vi "Read Pin Map.vi"(8 "error in (no error)":errorcluster, 11 "NI-DAQ in":refnum<class "NI-DAQ.lvclass">) -> (0 "error out":errorcluster, 2 "Pin Map":T1={"Region Valves"=[49, 52, 0, 0], "Extra Valves"=[[[0.0, 48.0, 0.0, 0.0, 0.0]]], "Tool Primary Valve"=51, "Tool Secondary Valve"=50, "Region Sensors"=[37, 41, 37], "Extra Sensors"=[[[36.0, 37.0, 0.0, 0.0]]], "Tool Primary Sensor"=39.0, "Tool Secondary Sensor"=38.0, "Compression Sensor"=31.0, "5V"=50}, 3 "NI-DAQ out":refnum<class "NI-DAQ.lvclass">)   [LabVIEW 2016, in "NI-DAQ.lvclass"]
uses:
  NI-DAQ.lvclass
  Pin Map.ctl
  I-O.lvclass
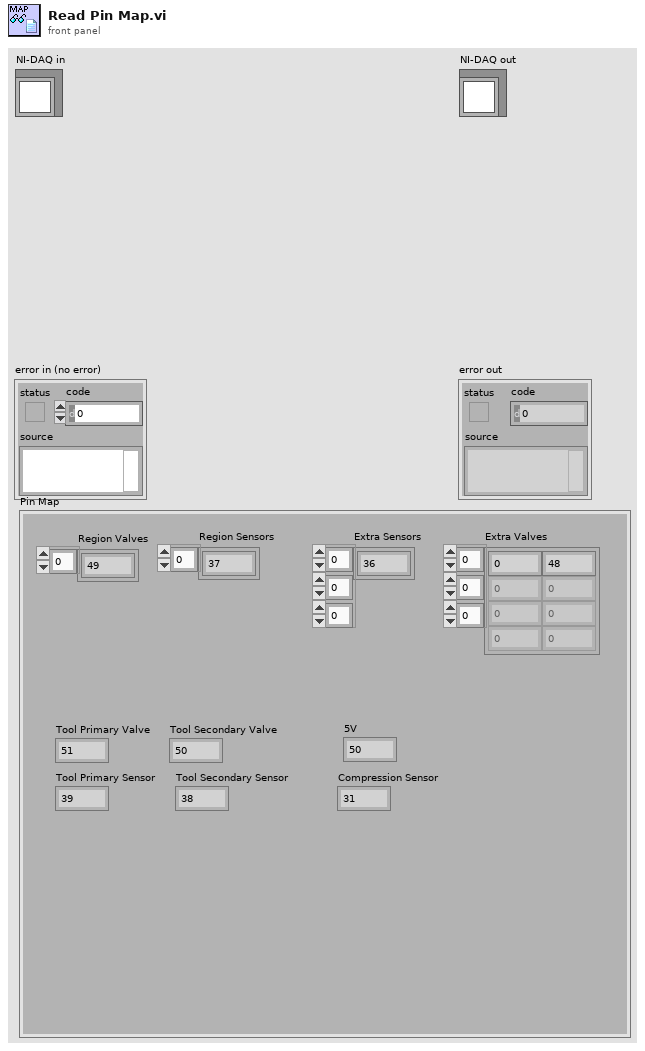
[diagram p1: front panel]
types:
  T1 = typedef "I-O.lvclass/Pin Map.ctl" = cluster{"Region Valves":i32[], "Extra Valves":dbl[][][], "Tool Primary Valve":i32, "Tool Secondary Valve":i32, "Region Sensors":i32[], "Extra Sensors":dbl[][][], "Tool Primary Sensor":dbl, "Tool Secondary Sensor":dbl, "Compression Sensor":dbl, "5V":i32}
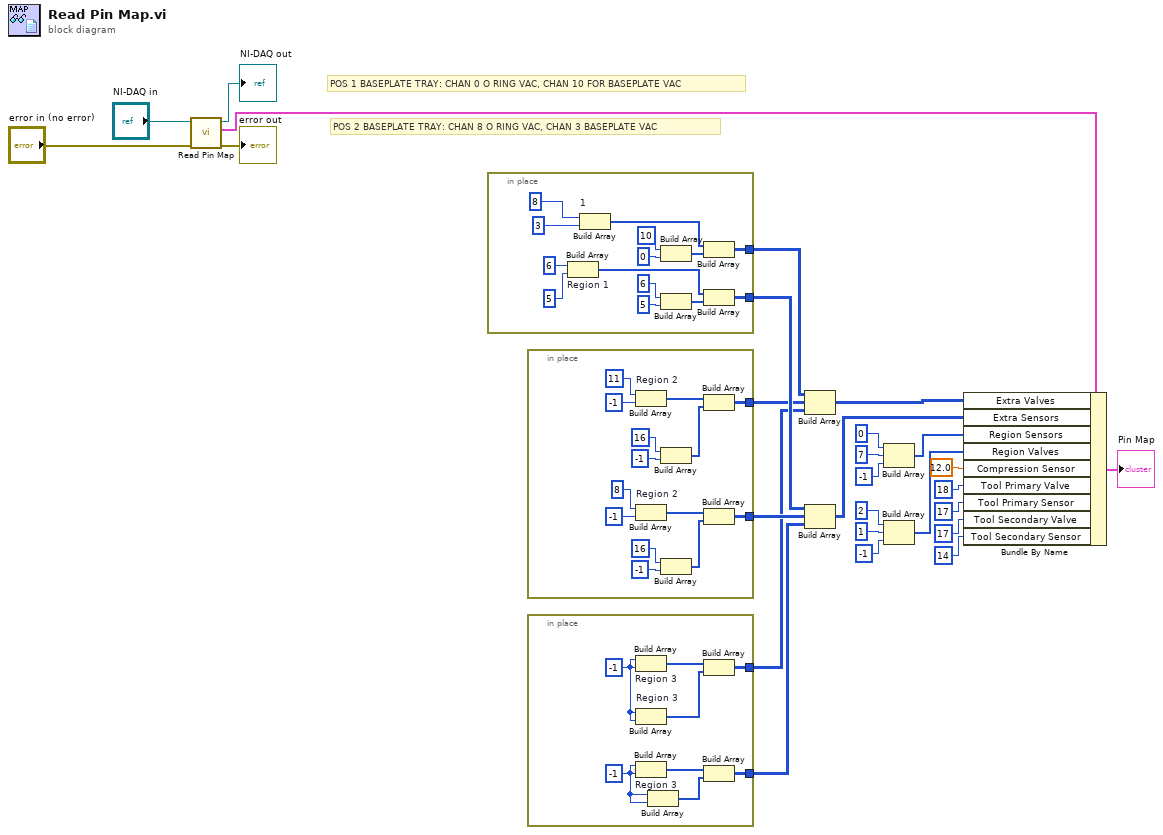
[diagram p0: block diagram]
diagram:
  # "POS 2 BASEPLATE TRAY: CHAN 8 O RING VAC, CHAN 3 BASEPLATE VAC"
  # "POS 1 BASEPLATE TRAY: CHAN 0 O RING VAC, CHAN 10 FOR BASEPLATE VAC"
  n1 = call-parent "Read Pin Map.vi"("error in (no error)"="error in (no error)", "I-O in"="NI-DAQ in") -> ("error out"=→"error out":errorcluster, "Pin Map"=w23:T1, "I-O out"=→"NI-DAQ out":refnum<class "NI-DAQ.lvclass">)  [unwired: 7 in]
  n2 = in-place {
    in-place-border: [w28] -> w8
    in-place-border: [w33] -> w3
    n3 = Build Array "Region 1"(6, 5 ("element")) -> (w30:i32[])
    n4 = Build Array "1"(8, 3 ("element")) -> (w35:i32[])
    n5 = Build Array(10, 0) -> (w34:i32[])
    n6 = Build Array(6 ("element"), 5 ("element")) -> (w29:i32[])
    n7 = Build Array(w35, w34) -> (w33:i32[][])
    n8 = Build Array(w30, w29) -> (w28:i32[][])
  }
  n9 = in-place {
    in-place-border: [w47] -> w7
    in-place-border: [w42] -> w6
    n10 = Build Array "Region 2"(11, -1) -> (w49:i32[])
    n11 = Build Array "Region 2"(8, -1 ("element")) -> (w44:i32[])
    n12 = Build Array(16 ("element"), -1) -> (w48:i32[])
    n13 = Build Array(16, -1 ("element")) -> (w43:i32[])
    n14 = Build Array(w49, w48) -> (w47:i32[][])
    n15 = Build Array(w44, w43) -> (w42:i32[][])
  }
  n16 = in-place {
    in-place-border: [w56] -> w5
    in-place-border: [w60] -> w4
    w59 = -1
    w63 = -1
    n17 = Build Array "Region 3"(w63, w63) -> (w62:i32[])
    n18 = Build Array "Region 3"(w63, w63) -> (w61:i32[])
    n19 = Build Array "Region 3"(w59, w59) -> (w58:i32[])
    n20 = Build Array(w59, w59) -> (w57:i32[])
    n21 = Build Array(w62, w61) -> (w60:i32[][])
    n22 = Build Array(w58, w57) -> (w56:i32[][])
  }
  n23 = Build Array(w3, w7, w4) -> (w2:i32[][][])
  n24 = Build Array(w8, w6, w5) -> (w1:i32[][][])
  n25 = Build Array(0, 7, -1) -> (w9:i32[])
  n26 = Build Array(2, 1, -1) -> (w15:i32[])
  n27 = Bundle By Name(cluster=w23, "Extra Valves"=w2, "Extra Sensors"=w1, "Region Sensors"=w9, "Region Valves"=w15, "Compression Sensor"=12.0, "Tool Primary Valve"=18, "Tool Primary Sensor"=17 ("Tool Primary Valve"), "Tool Secondary Valve"=17 ("Tool Primary Valve"), "Tool Secondary Sensor"=14 ("Tool Secondary Valve")) -> (→"Pin Map":T1)
